vi "_Parse ACLR NR Result.vi"(8 "error in (no error)":errorcluster, 10 "Input String":string, 11 "VISA resource name":refnum<visa-resource-name>) -> (0 "error out":errorcluster, 1 "ACLR Results":T1 {"NR Positive" format="%^.3e"; "NR Negative" format="%^.3e"; "UTRA 2 Positive" format="%^.3e"; "UTRA 1 Positive" format="%^.3e"; "Carrier" format="%^.3e"; "UTRA 1 Negative" format="%^.3e"; "UTRA 2 Negative" format="%^.3e"}, 2 "Reliability":i32, 3 "VISA resource name out":refnum<visa-resource-name>)   [LabVIEW 2020, in "Rohde&Schwarz CMWXP NR FR1 Measurement.lvlib"]
uses:
  <instrlib>/Rohde&Schwarz CMWXP NR FR1 Measurement/Rohde&Schwarz CMWXP NR FR1 Measurement.lvlib
  <instrlib>/Rohde&Schwarz CMWXP NR FR1 Measurement/Private/rsidr_core.llb/rsidr_core.lvlib
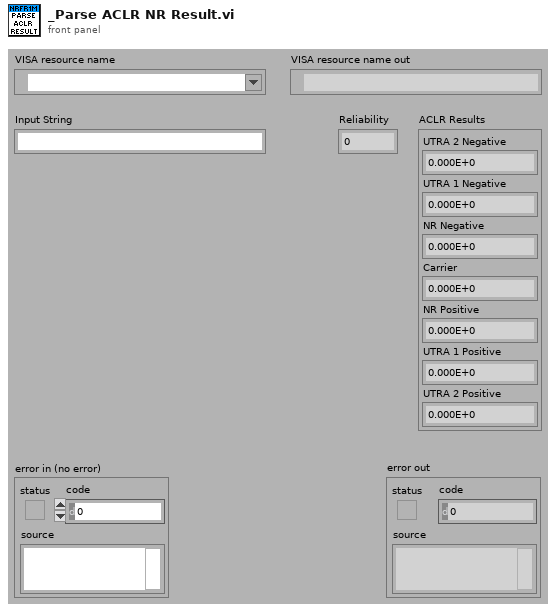
[diagram p1: front panel]
types:
  T1 = cluster{"UTRA 2 Negative":dbl, "UTRA 1 Negative":dbl, "NR Negative":dbl, "Carrier":dbl, "NR Positive":dbl, "UTRA 1 Positive":dbl, "UTRA 2 Positive":dbl}
  T2 = cluster{"double array out[0]":dbl, "double array out[1]":dbl, "double array out[2]":dbl, "double array out[3]":dbl, "double array out[4]":dbl, "double array out[5]":dbl, "double array out[6]":dbl}
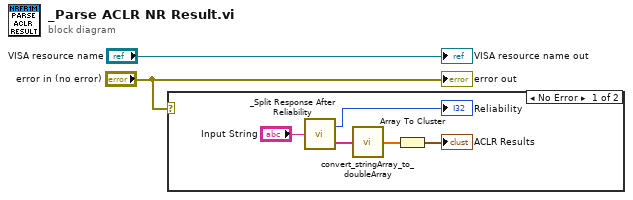
[diagram p0: block diagram]
diagram:
  n1 = case shown="No Error" "error in (no error)" {
    frame No Error {
      n2 = call <instrlib>:"_Split Response After Reliability.vi"("Input String"="Input String") -> ("Response out"=w5:string[], "Reliability out"=→"Reliability":i32)
      n3 = call <instrlib>:"convert_stringArray_to_doubleArray.vi"("string array in"=w5) -> ("double array out"=w4:dbl[])  [unwired: 4 in]
      n4 = Array To Cluster(array=w4) -> (cluster=→"ACLR Results":T2)
    }
    frame Error {
    }
  }
  "error out" <- "error in (no error)"
  "VISA resource name out" <- "VISA resource name"
